vi "Pre-Build Action.vi"(6 "Top Level/Always Included VIs":path[](array[path]), 7 "Main Destination Path":path, 9 "Target Name":string, 10 "Build Specification Name":string, 11 "Project Path":path) -> (0 "error out":errorcluster)   [LabVIEW 2023]
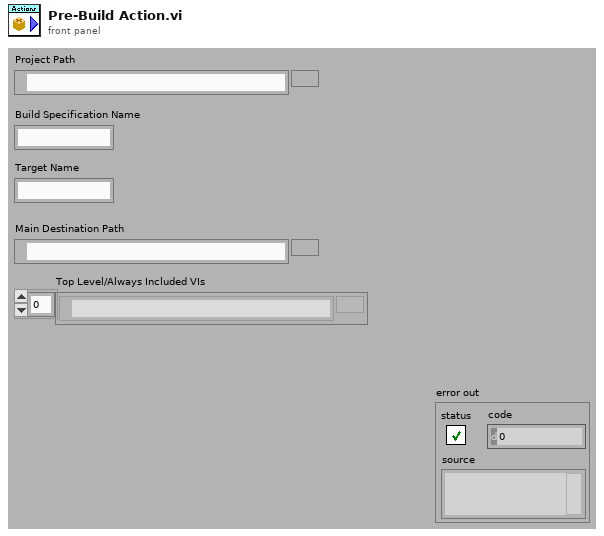
[diagram p1: front panel]
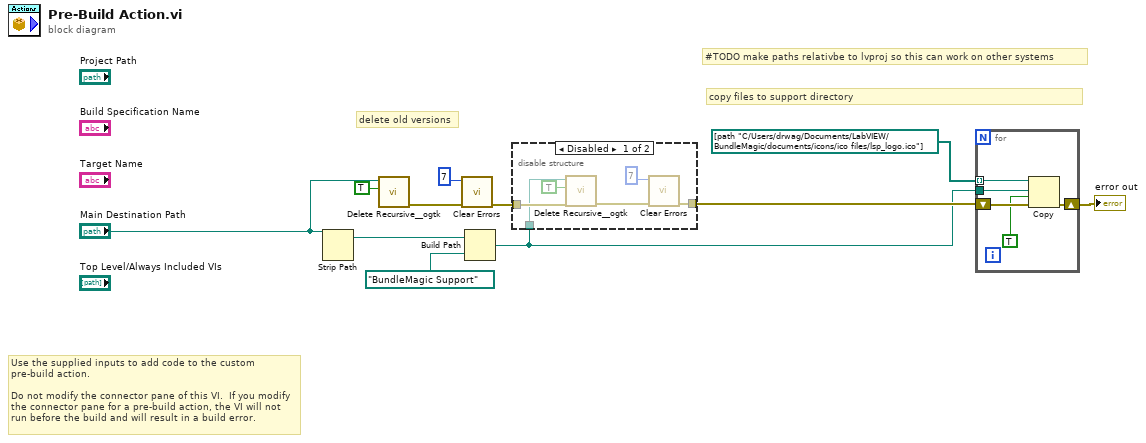
[diagram p0: block diagram]
diagram:
  # "#TODO make paths relativbe to lvproj so this can work on other systems"
  # "copy files to support directory"
  # "delete old versions"
  # "Use the supplied inputs to add code to the custom pre-build action.\n\nDo not modify the connector pane of this VI.  If you modify the connector pane for a pre-build action, the VI will not run before the build and will result in a build error."
  n1 = Strip Path(path="Main Destination Path") -> (stripped path=w9:path)  [unwired: 1 out]
  n2 = call <userlib>:"Delete Recursive__ogtk.vi"("Recursive? (FALSE)"=TRUE, "Path"="Main Destination Path") -> ("error out"=w8:errorcluster)  [unwired: 8 in, 1 out]
  n3 = call <vilib>:"Clear Errors.vi"("error in (no error)"=w8, "specific error code to clear (0: all)"=7) -> ("error out"=w3:errorcluster)  [unwired: 4 in, 1 out]
  n4 = Build Path(base path=w9, name or relative path=path "BundleMagic Support") -> (appended path=w1:path)
  n5 = disable-structure shown="Disabled" {
    disable-tunnel: w3 -> [w15 _]
    disable-tunnel: [w13 _] -> w2
    disable-tunnel: w1 -> [w12 _]
    frame Disabled {
      n6 = call <userlib>:"Delete Recursive__ogtk.vi"("error in (no error)"=w15, "Recursive? (FALSE)"=TRUE, "Path"=w12) -> ("error out"=w14:errorcluster)  [unwired: 7 in, 1 out]
      n7 = call <vilib>:"Clear Errors.vi"("error in (no error)"=w14, "specific error code to clear (0: all)"=7) -> ("error out"=w13:errorcluster)  [unwired: 4 in, 1 out]
    }
    frame Enabled {
    }
  }
  n8 = for {
    shift-right: [w21] -> w5
    shift-left: w2 -> [w22]
    tunnel: path[] [path "C:/Users/drwag/Documents/LabVIEW/BundleMagic/documents/icons/ico files/lsp_logo.ico"] ("name or relative path") -> [w20] mode=indexing
    tunnel: w1 -> [w19]
    n9 = Copy(8:w22, 9:TRUE ("overwrite (F)"), 10:w19, 11:w20) -> (0:w21:errorcluster)  [unwired: 1 in, 2 out]
  }
  "error out" <- w5
